vi "From Serial Form.vi"(6 "Serial Version":T1, 10 "Deserializer in":refnum<class "Deserializer.lvclass">, 11 "Data in":refnum<class "Data.lvclass">) -> (0 "error out":errorcluster, 2 "Deserializer out":refnum<class "Deserializer.lvclass">, 3 "Data out":refnum<class "Data.lvclass">)   [LabVIEW 2014, in "Base Data Class.lvlib" / "Data.lvclass"]
uses:
  Data.lvclass
  <vilib>/NI/AQ Character Lineator/Deserializer/Deserializer.lvclass
  <vilib>/NI/AQ Character Lineator/Serialization Common/Serial Version.ctl
  Data.lvclass/Data.ctl
  <vilib>/NI/AQ Character Lineator/Serializable/Remove Timestamp.vi
  <vilib>/NI/AQ Character Lineator/Serializable/Serializable.lvclass
  <vilib>/NI/AQ Character Lineator/Serialization Common/Serialization Common.lvlib
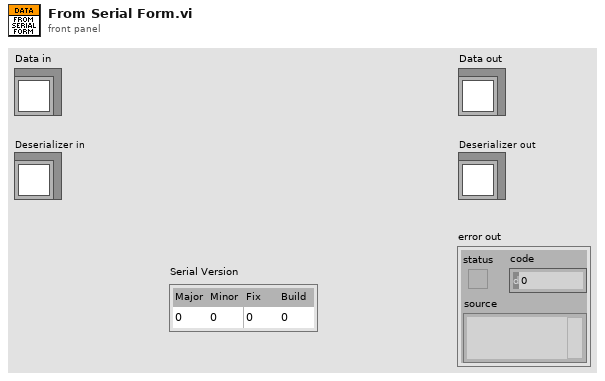
[diagram p1: front panel]
types:
  T1 = typedef "Serialization Common.lvlib/Serial Version.ctl" = cluster{"Major":u16, "Minor":u16, "Fix":u16, "Build":u16}
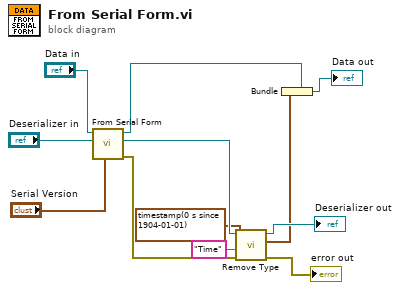
[diagram p0: block diagram]
diagram:
  n1 = call-parent "From Serial Form.vi"("Serial Version"="Serial Version", "Deserializer in"="Deserializer in", "Serializable in"="Data in") -> ("error out"=w8:errorcluster, "Deserializer out"=w9:refnum<class "Deserializer.lvclass">, "Serializable out"=w3:refnum<class "Data.lvclass">)  [unwired: 6 in]
  n2 = call-poly <vilib>:"Remove Type.vi"("error in (no error)"=w8, "Name"="Time", "Default Value"=timestamp(0 s since 1904-01-01), "Deserializer in"=w9) -> ("error out"=→"error out":errorcluster, "Time Stamp"=w2:timestamp, "Deserializer out"=→"Deserializer out":refnum<class "Deserializer.lvclass">)  [unwired: 4 in, 1 out]
  n3 = Bundle(cluster=w3, w2) -> (→"Data out":refnum<class "Data.lvclass">)
